vi "Vis-Prototype-ForceDirectedGraph-VIStaticLinkages.vi"() -> ()   [LabVIEW 2012]
uses:
  Dependencies/aws/AWS Shared/AWS-Shared-MetadataKeyValuePair.ctl
  Dependencies/aws/S3 API/AWS-S3-API.lvclass
panel:
  in  "Local Folder":path caption="(All output files will be copied to this location, old data may be overwritten!)"
  in  "Tab Control":T1(tab)=enum."HTML Page to Upload"
  in  "Local/Remote":string(combo)="Local"
  in  "S3 Bucket":string="visualize.wirebirdlabs.com" caption="(Default val provided merely as a convenience; feel free to output HTML/JSON to any local or remote server)"
  in  "Subfolder":string="gregSandbox" caption="(e.g., a subfolder \"mysandbox\" would upload to \"http://visualize.wirebirdlabs.com/mysandbox\")"
  in  "Access Key":string="AKIAJC4GLICEUISMCDHA"
  in  "Secret Key":string="WE0QzSnluCM5zp8GCpvH/PyVYhl7sW4CbsywKoKf"
  in  "Top-Level LabVIEW File (VI, LVClass, LVLib)":path caption="(e.g., drag the icon of this VI to this path control to scrape static linkages of itself)"
  in  "HTML Page":string="<!DOCTYPE HTML>\n<html dir=\"ltr\" lang=\"en-US\">\n\n<head>\n\n\t<!-- Title -->\n\t<title>VI Static Linkages as a Force-Directed Graph</title>\n\t\n\t<!-- SEO -->\n\t<meta name=\"robots\" content=\"noindex,noarchive,nosnippet\" />\n\n\t<!-- Stylesheets -->\n <link rel=\"stylesheet\" type=\"text/css\" media=\"all\" href=\"http://deploy.wirebirdlabs.com/Resources/Bootstrap/css/bootstrap.min.css\" />\n\t<link rel=\"stylesheet\" type=\"text/css\" media=\"all\" href=\"http://deploy.wirebirdlabs.com/Resources/FontAwesome/css/font-awesome.min.css\" />\n\t<link rel=\"stylesheet\" type=\"text/css\" media=\"all\" href=\"http://deploy.wirebirdlabs.com/Resources/Themes/Default/style.css\" />\n \n\t<!-- Scripts -->\n <script type='text/javascript' src='https://ajax.googleapis.com/ajax/libs/jquery/1.8.2/jquery.min.js'></script>\n\t<script type='text/javascript' src='http://deploy.wirebirdlabs.com/Resources/Bootstrap/js/bootstrap.min.js'></script>\n <script src=\"http://d3js.org/d3.v3.min.js\" charset=\"utf-8\"></script>\n\n\n <!-- Static Style Definitions -->\n <style>\n     .node {opacity: 0.5;}\n     .node:hover {opacity: 1;}\n     .node:not(:hover) text {display:none;}\n     .link {stroke: #999; stroke-opacity: 0.3;}\n</style>\n\n</head>\n\n<body class=\"container page-background\">\n\n\t<div class=\"container page-canvas\">\n\t\t<div class=\"page-header\">\n\t\t\t<h1 class=\"page-title page-title-title\">VI Static Linkages as a Force-Directed Graph</h1>\n\t\t</div>\n\n  <div class=\"page-body\">\n<div class=\"accordion\" id=\"legend\">\n  <div class=\"accordion-group template\">\n    <div class=\"accordion-heading\">\n        <a class=\"accordion-toggle\" data-toggle=\"collapse\" data-parent=\"#legend\" href=\"#collapseThree\">\n        </a>\n    </div>\n    <div id=\"collapseThree\" class=\"accordion-body collapse\">\n      <div class=\"accordion-inner\">\n      </div>\n    </div>\n  </div>\n</div>\n <!-- Begin code from http://bl.ocks.org/couchand/6420534 -->\n<div id=\"viz\"></div>\n <script>\n\nfunction name(d) { return d.name; }\nfunction group(d) { return d.group; }\n\nvar color = d3.scale.category10();\nfunction colorByGroup(d) { return color(group(d)); }\n\nvar width = <!-- Container-Width -->,\n    height = 960;\n\nvar svg = d3.select('#viz')\n    .append('svg')\n    .attr('width', width)\n    .attr('height', height);\n\nvar node, link;\n\nvar voronoi = d3.geom.voronoi()\n    .x(function(d) { return d.x; })\n    .y(function(d) { return d.y; })\n    .clipExtent([[-10, -10], [width+10, height+10]]);\n\nfunction recenterVoronoi(nodes) {\n    var shapes = [];\n    voronoi(nodes).forEach(function(d) {\n        if ( !d.length ) return;\n        var n = [];\n        d.forEach(function(c){\n            n.push([ c[0] - d.point.x, c[1] - d.point.y ]);\n        });\n        n.point = d.point;\n        shapes.push(n);\n    });\n    return shapes;\n}\n\nvar force = d3.layout.force()\n    .charge(-2000)\n    .friction(0.3)\n    .linkDistance(50)\n    .size([width, height]);\n\nforce.on('tick', function() {\n    node.attr('transform', function(d) { return 'translate('+d.x+','+d.y+')'; })\n        .attr('clip-path', function(d) { return 'url(#clip-'+d.index+')'; });\n\n    link.attr('x1', function(d) { return d.source.x; })\n        .attr('y1', function(d) { return d.source.y; })\n        .attr('x2', function(d) { return d.target.x; })\n        .attr('y2', function(d) { return d.target.y; });\n\n    var clip = svg.selectAll('.clip')\n        .data( recenterVoronoi(node.data()), function(d) { return d.point.index; } );\n\n    clip.enter().append('clipPath')\n        .attr('id', function(d) { return 'clip-'+d.point.index; })\n        .attr('class', 'clip');\n    clip.exit().remove()\n\n    clip.selectAll('path').remove();\n    clip.append('path')\n        .attr('d', function(d) { return 'M'+d.join(',')+'Z'; });\n});\n\nd3.json('root/static-linkages.json', function(err, data) {\n\n    data.nodes.forEach(function(d, i) {\n        d.id = i;\n    });\n\n    link = svg.selectAll('.link')\n        .data( data.links )\n      .enter().append('line')\n        .attr('class', 'link')\n        .style(\"stroke-width\", function(d) { return Math.sqrt(d.value); });\n\n    node = svg.selectAll('.node')\n        .data( data.nodes )\n      .enter().append('g')\n        .attr('title', name)\n        .attr('class', 'node')\n        .call( force.drag );\n\n    node.append('circle')\n        .attr('r', 30)\n        .attr('fill', colorByGroup)\n        .attr('fill-opacity', 0.5);\n\n    node.append('circle')\n        .attr('r', 4)\n        .attr('stroke', 'black');\n\n    node.append('text')\n        .text(function(d){return d.name;});\n\n    force\n        .nodes( data.nodes )\n        .links( data.links )\n        .start();\n\n\nvar $template = $(\".template\");\nvar names = new Array();\nnames = data.nodes;\nvar groupList = new Array();\n\n    function sortByKey(array, key) {\n    return array.sort(function(a, b) {\n        var x = a[key]; var y = b[key];\n        return ((x < y) ? -1 : ((x > y) ? 1 : 0));\n    });\n}\n\nsortByKey(names,'group');\n$.each(names, function(i,name) {\n    if (name.group != null && groupList.indexOf(name.group) < 0){\n    var $newPanel = $template.clone();\n    $newPanel.find(\".collapse\").removeClass(\"in\");\n    $newPanel.find(\".accordion-toggle\").attr(\"href\",  \"#\" + (name.group))\n             .text(\"Group #\" + name.group);\n    $newPanel.find(\".accordion-body\").attr(\"id\", name.group).addClass(\"collapse\").removeClass(\"in\");\n    $(\"#legend\").append($newPanel.fadeIn());\n    groupList.push(name.group);\n    }  \n$('#' + name.group).find('.accordion-inner').append(\"<p>\" + name.name + \"</p>\");\n});\n\nvar sortedLists;\n$.each(groupList,function(i,group){\n    var paragraphContent = $('#' + group).find('.accordion-inner p').get();\n    sortedLists = paragraphContent.sort(function(a, b){return ($(b).text().toUpperCase()) < ($(a).text().toUpperCase()) ? 1 : -1;})\n    $('#' + group).find('.accordion-inner').append(sortedLists);})\n\n});\n\n    </script>\n <!-- End code from http://bl.ocks.org/couchand/6420534 -->\n\n\t\t  <div class=\"page-footer row-fluid\">\n\t\t   \t<span class=\"span12\"></span>\n\t\t  </div>\n  </div>\n\t</div>\n\n\t<footer class=\"\">\n\t\t<p class=\"page-copyright\">Powered by: Friday nites and Halloween candy</p>\n\t\t<!-- Bootstrap Scripts -->\n\t\t<script type='text/javascript'>\n\t\t\tjQuery(document).ready( function(){\n\t\t\t\tjQuery('*[rel=popover]').popover();\n\t\t\t\tjQuery('*[rel=tooltip]').tooltip();} );\n\t\t</script>\n\t</footer>\n</body>\n</html>"
  in  "Default Data from http://bl.ocks.org/couchand/6420534":string="{\n  \"nodes\":[\n    {\"name\":\"Myriel\",\"group\":1},\n    {\"name\":\"Napoleon\",\"group\":1},\n    {\"name\":\"Mlle.Baptistine\",\"group\":1},\n    {\"name\":\"Mme.Magloire\",\"group\":1},\n    {\"name\":\"CountessdeLo\",\"group\":1},\n    {\"name\":\"Geborand\",\"group\":1},\n    {\"name\":\"Champtercier\",\"group\":1},\n    {\"name\":\"Cravatte\",\"group\":1},\n    {\"name\":\"Count\",\"group\":1},\n    {\"name\":\"OldMan\",\"group\":1},\n    {\"name\":\"Labarre\",\"group\":2},\n    {\"name\":\"Valjean\",\"group\":2},\n    {\"name\":\"Marguerite\",\"group\":3},\n    {\"name\":\"Mme.deR\",\"group\":2},\n    {\"name\":\"Isabeau\",\"group\":2},\n    {\"name\":\"Gervais\",\"group\":2},\n    {\"name\":\"Tholomyes\",\"group\":3},\n    {\"name\":\"Listolier\",\"group\":3},\n    {\"name\":\"Fameuil\",\"group\":3},\n    {\"name\":\"Blacheville\",\"group\":3},\n    {\"name\":\"Favourite\",\"group\":3},\n    {\"name\":\"Dahlia\",\"group\":3},\n    {\"name\":\"Zephine\",\"group\":3},\n    {\"name\":\"Fantine\",\"group\":3},\n    {\"name\":\"Mme.Thenardier\",\"group\":4},\n    {\"name\":\"Thenardier\",\"group\":4},\n    {\"name\":\"Cosette\",\"group\":5},\n    {\"name\":\"Javert\",\"group\":4},\n    {\"name\":\"Fauchelevent\",\"group\":0},\n    {\"name\":\"Bamatabois\",\"group\":2},\n    {\"name\":\"Perpetue\",\"group\":3},\n    {\"name\":\"Simplice\",\"group\":2},\n    {\"name\":\"Scaufflaire\",\"group\":2},\n    {\"name\":\"Woman1\",\"group\":2},\n    {\"name\":\"Judge\",\"group\":2},\n    {\"name\":\"Champmathieu\",\"group\":2},\n    {\"name\":\"Brevet\",\"group\":2},\n    {\"name\":\"Chenildieu\",\"group\":2},\n    {\"name\":\"Cochepaille\",\"group\":2},\n    {\"name\":\"Pontmercy\",\"group\":4},\n    {\"name\":\"Boulatruelle\",\"group\":6},\n    {\"name\":\"Eponine\",\"group\":4},\n    {\"name\":\"Anzelma\",\"group\":4},\n    {\"name\":\"Woman2\",\"group\":5},\n    {\"name\":\"MotherInnocent\",\"group\":0},\n    {\"name\":\"Gribier\",\"group\":0},\n    {\"name\":\"Jondrette\",\"group\":7},\n    {\"name\":\"Mme.Burgon\",\"group\":7},\n    {\"name\":\"Gavroche\",\"group\":8},\n    {\"name\":\"Gillenormand\",\"group\":5},\n    {\"name\":\"Magnon\",\"group\":5},\n    {\"name\":\"Mlle.Gillenormand\",\"group\":5},\n    {\"name\":\"Mme.Pontmercy\",\"group\":5},\n    {\"name\":\"Mlle.Vaubois\",\"group\":5},\n    {\"name\":\"Lt.Gillenormand\",\"group\":5},\n    {\"name\":\"Marius\",\"group\":8},\n    {\"name\":\"BaronessT\",\"group\":5},\n    {\"name\":\"Mabeuf\",\"group\":8},\n    {\"name\":\"Enjolras\",\"group\":8},\n    {\"name\":\"Combeferre\",\"group\":8},\n    {\"name\":\"Prouvaire\",\"group\":8},\n    {\"name\":\"Feuilly\",\"group\":8},\n    {\"name\":\"Courfeyrac\",\"group\":8},\n    {\"name\":\"Bahorel\",\"group\":8},\n    {\"name\":\"Bossuet\",\"group\":8},\n    {\"name\":\"Joly\",\"group\":8},\n    {\"name\":\"Grantaire\",\"group\":8},\n    {\"name\":\"MotherPlutarch\",\"group\":9},\n    {\"name\":\"Gueulemer\",\"group\":4},\n    {\"name\":\"Babet\",\"group\":4},\n    {\"name\":\"Claquesous\",\"group\":4},\n    {\"name\":\"Montparnasse\",\"group\":4},\n    {\"name\":\"Toussaint\",\"group\":5},\n    {\"name\":\"Child1\",\"group\":10},\n    {\"name\":\"Child2\",\"group\":10},\n    {\"name\":\"Brujon\",\"group\":4},\n    {\"name\":\"Mme.Hucheloup\",\"group\":8}\n  ],\n  \"links\":[\n    {\"source\":1,\"target\":0,\"value\":1},\n    {\"source\":2,\"target\":0,\"value\":8},\n    {\"source\":3,\"target\":0,\"value\":10},\n    {\"source\":3,\"target\":2,\"value\":6},\n    {\"source\":4,\"target\":0,\"value\":1},\n    {\"source\":5,\"target\":0,\"value\":1},\n    {\"source\":6,\"target\":0,\"value\":1},\n    {\"source\":7,\"target\":0,\"value\":1},\n    {\"source\":8,\"target\":0,\"value\":2},\n    {\"source\":9,\"target\":0,\"value\":1},\n    {\"source\":11,\"target\":10,\"value\":1},\n    {\"source\":11,\"target\":3,\"value\":3},\n    {\"source\":11,\"target\":2,\"value\":3},\n    {\"source\":11,\"target\":0,\"value\":5},\n    {\"source\":12,\"target\":11,\"value\":1},\n    {\"source\":13,\"target\":11,\"value\":1},\n    {\"source\":14,\"target\":11,\"value\":1},\n    {\"source\":15,\"target\":11,\"value\":1},\n    {\"source\":17,\"target\":16,\"value\":4},\n    {\"source\":18,\"target\":16,\"value\":4},\n    {\"source\":18,\"target\":17,\"value\":4},\n    {\"source\":19,\"target\":16,\"value\":4},\n    {\"source\":19,\"target\":17,\"value\":4},\n    {\"source\":19,\"target\":18,\"value\":4},\n    {\"source\":20,\"target\":16,\"value\":3},\n    {\"source\":20,\"target\":17,\"value\":3},\n    {\"source\":20,\"target\":18,\"value\":3},\n    {\"source\":20,\"target\":19,\"value\":4},\n    {\"source\":21,\"target\":16,\"value\":3},\n    {\"source\":21,\"target\":17,\"value\":3},\n    {\"source\":21,\"target\":18,\"value\":3},\n    {\"source\":21,\"target\":19,\"value\":3},\n    {\"source\":21,\"target\":20,\"value\":5},\n    {\"source\":22,\"target\":16,\"value\":3},\n    {\"source\":22,\"target\":17,\"value\":3},\n    {\"source\":22,\"target\":18,\"value\":3},\n    {\"source\":22,\"target\":19,\"value\":3},\n    {\"source\":22,\"target\":20,\"value\":4},\n    {\"source\":22,\"target\":21,\"value\":4},\n    {\"source\":23,\"target\":16,\"value\":3},\n    {\"source\":23,\"target\":17,\"value\":3},\n    {\"source\":23,\"target\":18,\"value\":3},\n    {\"source\":23,\"target\":19,\"value\":3},\n    {\"source\":23,\"target\":20,\"value\":4},\n    {\"source\":23,\"target\":21,\"value\":4},\n    {\"source\":23,\"target\":22,\"value\":4},\n    {\"source\":23,\"target\":12,\"value\":2},\n    {\"source\":23,\"target\":11,\"value\":9},\n    {\"source\":24,\"target\":23,\"value\":2},\n    {\"source\":24,\"target\":11,\"value\":7},\n    {\"source\":25,\"target\":24,\"value\":13},\n    {\"source\":25,\"target\":23,\"value\":1},\n    {\"source\":25,\"target\":11,\"value\":12},\n    {\"source\":26,\"target\":24,\"value\":4},\n    {\"source\":26,\"target\":11,\"value\":31},\n    {\"source\":26,\"target\":16,\"value\":1},\n    {\"source\":26,\"target\":25,\"value\":1},\n    {\"source\":27,\"target\":11,\"value\":17},\n    {\"source\":27,\"target\":23,\"value\":5},\n    {\"source\":27,\"target\":25,\"value\":5},\n    {\"source\":27,\"target\":24,\"value\":1},\n    {\"source\":27,\"target\":26,\"value\":1},\n    {\"source\":28,\"target\":11,\"value\":8},\n    {\"source\":28,\"target\":27,\"value\":1},\n    {\"source\":29,\"target\":23,\"value\":1},\n    {\"source\":29,\"target\":27,\"value\":1},\n    {\"source\":29,\"target\":11,\"value\":2},\n    {\"source\":30,\"target\":23,\"value\":1},\n    {\"source\":31,\"target\":30,\"value\":2},\n    {\"source\":31,\"target\":11,\"value\":3},\n    {\"source\":31,\"target\":23,\"value\":2},\n    {\"source\":31,\"target\":27,\"value\":1},\n    {\"source\":32,\"target\":11,\"value\":1},\n    {\"source\":33,\"target\":11,\"value\":2},\n    {\"source\":33,\"target\":27,\"value\":1},\n    {\"source\":34,\"target\":11,\"value\":3},\n    {\"source\":34,\"target\":29,\"value\":2},\n    {\"source\":35,\"target\":11,\"value\":3},\n    {\"source\":35,\"target\":34,\"value\":3},\n    {\"source\":35,\"target\":29,\"value\":2},\n    {\"source\":36,\"target\":34,\"value\":2},\n    {\"source\":36,\"target\":35,\"value\":2},\n    {\"source\":36,\"target\":11,\"value\":2},\n    {\"source\":36,\"target\":29,\"value\":1},\n    {\"source\":37,\"target\":34,\"value\":2},\n    {\"source\":37,\"target\":35,\"value\":2},\n    {\"source\":37,\"target\":36,\"value\":2},\n    {\"source\":37,\"target\":11,\"value\":2},\n    {\"source\":37,\"target\":29,\"value\":1},\n    {\"source\":38,\"target\":34,\"value\":2},\n    {\"source\":38,\"target\":35,\"value\":2},\n    {\"source\":38,\"target\":36,\"value\":2},\n    {\"source\":38,\"target\":37,\"value\":2},\n    {\"source\":38,\"target\":11,\"value\":2},\n    {\"source\":38,\"target\":29,\"value\":1},\n    {\"source\":39,\"target\":25,\"value\":1},\n    {\"source\":40,\"target\":25,\"value\":1},\n    {\"source\":41,\"target\":24,\"value\":2},\n    {\"source\":41,\"target\":25,\"value\":3},\n    {\"source\":42,\"target\":41,\"value\":2},\n    {\"source\":42,\"target\":25,\"value\":2},\n    {\"source\":42,\"target\":24,\"value\":1},\n    {\"source\":43,\"target\":11,\"value\":3},\n    {\"source\":43,\"target\":26,\"value\":1},\n    {\"source\":43,\"target\":27,\"value\":1},\n    {\"source\":44,\"target\":28,\"value\":3},\n    {\"source\":44,\"target\":11,\"value\":1},\n    {\"source\":45,\"target\":28,\"value\":2},\n    {\"source\":47,\"target\":46,\"value\":1},\n    {\"source\":48,\"target\":47,\"value\":2},\n    {\"source\":48,\"target\":25,\"value\":1},\n    {\"source\":48,\"target\":27,\"value\":1},\n    {\"source\":48,\"target\":11,\"value\":1},\n    {\"source\":49,\"target\":26,\"value\":3},\n    {\"source\":49,\"target\":11,\"value\":2},\n    {\"source\":50,\"target\":49,\"value\":1},\n    {\"source\":50,\"target\":24,\"value\":1},\n    {\"source\":51,\"target\":49,\"value\":9},\n    {\"source\":51,\"target\":26,\"value\":2},\n    {\"source\":51,\"target\":11,\"value\":2},\n    {\"source\":52,\"target\":51,\"value\":1},\n    {\"source\":52,\"target\":39,\"value\":1},\n    {\"source\":53,\"target\":51,\"value\":1},\n    {\"source\":54,\"target\":51,\"value\":2},\n    {\"source\":54,\"target\":49,\"value\":1},\n    {\"source\":54,\"target\":26,\"value\":1},\n    {\"source\":55,\"target\":51,\"value\":6},\n    {\"source\":55,\"target\":49,\"value\":12},\n    {\"source\":55,\"target\":39,\"value\":1},\n    {\"source\":55,\"target\":54,\"value\":1},\n    {\"source\":55,\"target\":26,\"value\":21},\n    {\"source\":55,\"target\":11,\"value\":19},\n    {\"source\":55,\"target\":16,\"value\":1},\n    {\"source\":55,\"target\":25,\"value\":2},\n    {\"source\":55,\"target\":41,\"value\":5},\n    {\"source\":55,\"target\":48,\"value\":4},\n    {\"source\":56,\"target\":49,\"value\":1},\n    {\"source\":56,\"target\":55,\"value\":1},\n    {\"source\":57,\"target\":55,\"value\":1},\n    {\"source\":57,\"target\":41,\"value\":1},\n    {\"source\":57,\"target\":48,\"value\":1},\n    {\"source\":58,\"target\":55,\"value\":7},\n    {\"source\":58,\"target\":48,\"value\":7},\n    {\"source\":58,\"target\":27,\"value\":6},\n    {\"source\":58,\"target\":57,\"value\":1},\n    {\"source\":58,\"target\":11,\"value\":4},\n    {\"source\":59,\"target\":58,\"value\":15},\n    {\"source\":59,\"target\":55,\"value\":5},\n    {\"source\":59,\"target\":48,\"value\":6},\n    {\"source\":59,\"target\":57,\"value\":2},\n    {\"source\":60,\"target\":48,\"value\":1},\n    {\"source\":60,\"target\":58,\"value\":4},\n    {\"source\":60,\"target\":59,\"value\":2},\n    {\"source\":61,\"target\":48,\"value\":2},\n    {\"source\":61,\"target\":58,\"value\":6},\n    {\"source\":61,\"target\":60,\"value\":2},\n    {\"source\":61,\"target\":59,\"value\":5},\n    {\"source\":61,\"target\":57,\"value\":1},\n    {\"source\":61,\"target\":55,\"value\":1},\n    {\"source\":62,\"target\":55,\"value\":9},\n    {\"source\":62,\"target\":58,\"value\":17},\n    {\"source\":62,\"target\":59,\"value\":13},\n    {\"source\":62,\"target\":48,\"value\":7},\n    {\"source\":62,\"target\":57,\"value\":2},\n    {\"source\":62,\"target\":41,\"value\":1},\n    {\"source\":62,\"target\":61,\"value\":6},\n    {\"source\":62,\"target\":60,\"value\":3},\n    {\"source\":63,\"target\":59,\"value\":5},\n    {\"source\":63,\"target\":48,\"value\":5},\n    {\"source\":63,\"target\":62,\"value\":6},\n    {\"source\":63,\"target\":57,\"value\":2},\n    {\"source\":63,\"target\":58,\"value\":4},\n    {\"source\":63,\"target\":61,\"value\":3},\n    {\"source\":63,\"target\":60,\"value\":2},\n    {\"source\":63,\"target\":55,\"value\":1},\n    {\"source\":64,\"target\":55,\"value\":5},\n    {\"source\":64,\"target\":62,\"value\":12},\n    {\"source\":64,\"target\":48,\"value\":5},\n    {\"source\":64,\"target\":63,\"value\":4},\n    {\"source\":64,\"target\":58,\"value\":10},\n    {\"source\":64,\"target\":61,\"value\":6},\n    {\"source\":64,\"target\":60,\"value\":2},\n    {\"source\":64,\"target\":59,\"value\":9},\n    {\"source\":64,\"target\":57,\"value\":1},\n    {\"source\":64,\"target\":11,\"value\":1},\n    {\"source\":65,\"target\":63,\"value\":5},\n    {\"source\":65,\"target\":64,\"value\":7},\n    {\"source\":65,\"target\":48,\"value\":3},\n    {\"source\":65,\"target\":62,\"value\":5},\n    {\"source\":65,\"target\":58,\"value\":5},\n    {\"source\":65,\"target\":61,\"value\":5},\n    {\"source\":65,\"target\":60,\"value\":2},\n    {\"source\":65,\"target\":59,\"value\":5},\n    {\"source\":65,\"target\":57,\"value\":1},\n    {\"source\":65,\"target\":55,\"value\":2},\n    {\"source\":66,\"target\":64,\"value\":3},\n    {\"source\":66,\"target\":58,\"value\":3},\n    {\"source\":66,\"target\":59,\"value\":1},\n    {\"source\":66,\"target\":62,\"value\":2},\n    {\"source\":66,\"target\":65,\"value\":2},\n    {\"source\":66,\"target\":48,\"value\":1},\n    {\"source\":66,\"target\":63,\"value\":1},\n    {\"source\":66,\"target\":61,\"value\":1},\n    {\"source\":66,\"target\":60,\"value\":1},\n    {\"source\":67,\"target\":57,\"value\":3},\n    {\"source\":68,\"target\":25,\"value\":5},\n    {\"source\":68,\"target\":11,\"value\":1},\n    {\"source\":68,\"target\":24,\"value\":1},\n    {\"source\":68,\"target\":27,\"value\":1},\n    {\"source\":68,\"target\":48,\"value\":1},\n    {\"source\":68,\"target\":41,\"value\":1},\n    {\"source\":69,\"target\":25,\"value\":6},\n    {\"source\":69,\"target\":68,\"value\":6},\n    {\"source\":69,\"target\":11,\"value\":1},\n    {\"source\":69,\"target\":24,\"value\":1},\n    {\"source\":69,\"target\":27,\"value\":2},\n    {\"source\":69,\"target\":48,\"value\":1},\n    {\"source\":69,\"target\":41,\"value\":1},\n    {\"source\":70,\"target\":25,\"value\":4},\n    {\"source\":70,\"target\":69,\"value\":4},\n    {\"source\":70,\"target\":68,\"value\":4},\n    {\"source\":70,\"target\":11,\"value\":1},\n    {\"source\":70,\"target\":24,\"value\":1},\n    {\"source\":70,\"target\":27,\"value\":1},\n    {\"source\":70,\"target\":41,\"value\":1},\n    {\"source\":70,\"target\":58,\"value\":1},\n    {\"source\":71,\"target\":27,\"value\":1},\n    {\"source\":71,\"target\":69,\"value\":2},\n    {\"source\":71,\"target\":68,\"value\":2},\n    {\"source\":71,\"target\":70,\"value\":2},\n    {\"source\":71,\"target\":11,\"value\":1},\n    {\"source\":71,\"target\":48,\"value\":1},\n    {\"source\":71,\"target\":41,\"value\":1},\n    {\"source\":71,\"target\":25,\"value\":1},\n    {\"source\":72,\"target\":26,\"value\":2},\n    {\"source\":72,\"target\":27,\"value\":1},\n    {\"source\":72,\"target\":11,\"value\":1},\n    {\"source\":73,\"target\":48,\"value\":2},\n    {\"source\":74,\"target\":48,\"value\":2},\n    {\"source\":74,\"target\":73,\"value\":3},\n    {\"source\":75,\"target\":69,\"value\":3},\n    {\"source\":75,\"target\":68,\"value\":3},\n    {\"source\":75,\"target\":25,\"value\":3},\n    {\"source\":75,\"target\":48,\"value\":1},\n    {\"source\":75,\"target\":41,\"value\":1},\n    {\"source\":75,\"target\":70,\"value\":1},\n    {\"source\":75,\"target\":71,\"value\":1},\n    {\"source\":76,\"target\":64,\"value\":1},\n    {\"source\":76,\"target\":65,\"value\":1},\n    {\"source\":76,\"target\":66,\"value\":1},\n    {\"source\":76,\"target\":63,\"value\":1},\n    {\"source\":76,\"target\":62,\"value\":1},\n    {\"source\":76,\"target\":48,\"value\":1},\n    {\"source\":76,\"target\":58,\"value\":1}\n  ]\n}"
  out "Status":string="Progress: 0049 of 0049"
  out "Nodes and Linkages":string="{\n\"nodes\":\n[    {\"name\":\"Vis-Prototype-ForceDirectedGraph-VIStaticLinkages.vi\",\"group\":2},\n     {\"name\":\"AWS-Shared-MetadataKeyValuePair.ctl\",\"group\":2},\n     {\"name\":\"WirebirdLabs-VIServer-LinkerInfo.vi\",\"group\":2},\n     {\"name\":\"WirebirdLabs-VIServer-LinkerInfoStructure.ctl\",\"group\":2},\n     {\"name\":\"FTW-JSON-Array-Serialize.vi\",\"group\":2},\n     {\"name\":\"WirebirdLabs-STR-DelimitStringArray.vi\",\"group\":2},\n     {\"name\":\"AWS-S3-API.lvclass:AWS-S3-ConstructClient.vi\",\"group\":1},\n     {\"name\":\"AWS-S3-API.lvclass\",\"group\":0},\n     {\"name\":\"AWS-S3-API.lvclass:AWS-S3-API.ctl\",\"group\":1},\n     {\"name\":\"mscorlib\",\"group\":4},\n     {\"name\":\"AWS-S3-API.lvclass:AWS-S3-Transfer-Progress.ctl\",\"group\":1},\n     {\"name\":\"AWS-S3-API.lvclass:AWS-S3-Transfer-Header.ctl\",\"group\":1},\n     {\"name\":\"AWS-S3-API.lvclass:AWS-S3-Transfer-Completed.ctl\",\"group\":1},\n     {\"name\":\"AWS-S3-API.lvclass:AWS-S3-ClientRef-Get.vi\",\"group\":1},\n     {\"name\":\"E:\\u005CWirebirdLabs\\u005CVisualize\\u005CDependencies\\u005Caws\\u005CAWS-SDK\\u005CAWSSDK.dll\",\"group\":4},\n     {\"name\":\"AWS-S3-API.lvclass:AWS-S3-ClientRef-Set.vi\",\"group\":1},\n     {\"name\":\"AWS-S3-API.lvclass:AWS-S3-ObjectURL.vi\",\"group\":1},\n     {\"name\":\"WirebirdLabs-ERR-Clear.vi\",\"group\":2},\n     {\"name\":\"AWS-S3-API.lvclass:AWS-S3-ProcessDownload.vi\",\"group\":1},\n     {\"name\":\"AWS-S3-API.lvclass:AWS-S3-ProcessUpload.vi\",\"group\":1},\n     {\"name\":\"AWS-S3-API.lvclass:AWS-S3-ProgressCallbackDownload.vi\",\"group\":1},\n     {\"name\":\"AWS-S3-API.lvclass:AWS-S3-SendProgressUpdate.vi\",\"group\":1},\n     {\"name\":\"AWS-S3-API.lvclass:AWS-S3-ProgressCallbackUpload.vi\",\"group\":1},\n     {\"name\":\"AWS-S3-API.lvclass:AWS-S3-BeginDownload.vi\",\"group\":1},\n     {\"name\":\"WirebirdLabs-Time-Timer.vi\",\"group\":2},\n     {\"name\":\"WirebirdLabs-VIServer-AsyncCallOptions.vi\",\"group\":2},\n     {\"name\":\"AWS-S3-API.lvclass:AWS-S3-BeginUpload.vi\",\"group\":1},\n     {\"name\":\"WirebirdLabs-File-FileInfo.vi\",\"group\":2},\n     {\"name\":\"FTW-STR-Display-Bytes.vi\",\"group\":2},\n     {\"name\":\"AWS-Shared-MD5ofFile.vi\",\"group\":2},\n     {\"name\":\"AWS-S3-API.lvclass:AWS-S3-BucketCreate.vi\",\"group\":1},\n     {\"name\":\"AWS-S3-API.lvclass:AWS-S3-BucketSetPolicy.vi\",\"group\":1},\n     {\"name\":\"AWS-S3-API.lvclass:AWS-S3-BucketSettings.vi\",\"group\":1},\n     {\"name\":\"AWS-S3-API.lvclass:AWS-S3-DestroyClient.vi\",\"group\":1},\n     {\"name\":\"AWS-S3-API.lvclass:AWS-S3-GenerateExpiringLink.vi\",\"group\":1},\n     {\"name\":\"AWS-S3-API.lvclass:AWS-S3-GetObjectData.vi\",\"group\":1},\n     {\"name\":\"AWS-S3-API.lvclass:AWS-S3-GetProgressEvent.vi\",\"group\":1},\n     {\"name\":\"AWS-S3-API.lvclass:AWS-S3-ListBuckets.vi\",\"group\":1},\n     {\"name\":\"AWS-S3-API.lvclass:AWS-S3-ListObjectsInBucket.vi\",\"group\":1},\n     {\"name\":\"System\",\"group\":4},\n     {\"name\":\"AWS-S3-API.lvclass:AWS-S3-PutObjectData.vi\",\"group\":1},\n     {\"name\":\"AWS-Shared-MD5ofContent.vi\",\"group\":2},\n     {\"name\":\"AWS-S3-API.lvclass:AWS-S3-SynchronousUpload.vi\",\"group\":1},\n     {\"name\":\"AWS-S3-API.lvclass:AWS-S3-Transfer-Abort.vi\",\"group\":1},\n     {\"name\":\"Get File Extension.vi\",\"group\":2},\n     {\"name\":\"C:\\u005CProgram Files (x86)\\u005CNational Instruments\\u005CLabVIEW 2012\\u005Chelp\\u005Cglang.chm\",\"group\":4},\n     {\"name\":\"FTW-JSON-Format-String.vi\",\"group\":2},\n     {\"name\":\"WirebirdLabs-JSON-Escape.vi\",\"group\":2},\n     {\"name\":\"Error Cluster From Error Code.vi\",\"group\":2}],\n\"links\":\n[    {\"source\":0,\"target\":1,\"value\":9},\n     {\"source\":0,\"target\":2,\"value\":9},\n     {\"source\":0,\"target\":4,\"value\":9},\n     {\"source\":0,\"target\":6,\"value\":9},\n     {\"source\":0,\"target\":40,\"value\":9},\n     {\"source\":0,\"target\":33,\"value\":9},\n     {\"source\":0,\"target\":44,\"value\":9},\n     {\"source\":0,\"target\":46,\"value\":9},\n     {\"source\":0,\"target\":48,\"value\":9},\n     {\"source\":2,\"target\":3,\"value\":1},\n     {\"source\":4,\"target\":5,\"value\":1},\n     {\"source\":6,\"target\":7,\"value\":7},\n     {\"source\":6,\"target\":10,\"value\":7},\n     {\"source\":6,\"target\":11,\"value\":7},\n     {\"source\":6,\"target\":12,\"value\":7},\n     {\"source\":6,\"target\":14,\"value\":7},\n     {\"source\":6,\"target\":8,\"value\":7},\n     {\"source\":6,\"target\":15,\"value\":7},\n     {\"source\":7,\"target\":8,\"value\":27},\n     {\"source\":7,\"target\":13,\"value\":27},\n     {\"source\":7,\"target\":15,\"value\":27},\n     {\"source\":7,\"target\":16,\"value\":27},\n     {\"source\":7,\"target\":18,\"value\":27},\n     {\"source\":7,\"target\":19,\"value\":27},\n     {\"source\":7,\"target\":20,\"value\":27},\n     {\"source\":7,\"target\":22,\"value\":27},\n     {\"source\":7,\"target\":21,\"value\":27},\n     {\"source\":7,\"target\":23,\"value\":27},\n     {\"source\":7,\"target\":26,\"value\":27},\n     {\"source\":7,\"target\":30,\"value\":27},\n     {\"source\":7,\"target\":31,\"value\":27},\n     {\"source\":7,\"target\":32,\"value\":27},\n     {\"source\":7,\"target\":6,\"value\":27},\n     {\"source\":7,\"target\":33,\"value\":27},\n     {\"source\":7,\"target\":34,\"value\":27},\n     {\"source\":7,\"target\":35,\"value\":27},\n     {\"source\":7,\"target\":36,\"value\":27},\n     {\"source\":7,\"target\":37,\"value\":27},\n     {\"source\":7,\"target\":38,\"value\":27},\n     {\"source\":7,\"target\":40,\"value\":27},\n     {\"source\":7,\"target\":42,\"value\":27},\n     {\"source\":7,\"target\":43,\"value\":27},\n     {\"source\":7,\"target\":12,\"value\":27},\n     {\"source\":7,\"target\":11,\"value\":27},\n     {\"source\":7,\"target\":10,\"value\":27},\n     {\"source\":8,\"target\":7,\"value\":5},\n     {\"source\":8,\"target\":9,\"value\":5},\n     {\"source\":8,\"target\":10,\"value\":5},\n     {\"source\":8,\"target\":11,\"value\":5},\n     {\"source\":8,\"target\":12,\"value\":5},\n     {\"source\":10,\"target\":7,\"value\":2},\n     {\"source\":10,\"target\":11,\"value\":2},\n     {\"source\":11,\"target\":7,\"value\":1},\n     {\"source\":12,\"target\":7,\"value\":2},\n     {\"source\":12,\"target\":11,\"value\":2},\n     {\"source\":13,\"target\":7,\"value\":3},\n     {\"source\":13,\"target\":14,\"value\":3},\n     {\"source\":13,\"target\":8,\"value\":3},\n     {\"source\":15,\"target\":7,\"value\":3},\n     {\"source\":15,\"target\":14,\"value\":3},\n     {\"source\":15,\"target\":8,\"value\":3},\n     {\"source\":16,\"target\":7,\"value\":2},\n     {\"source\":16,\"target\":17,\"value\":2},\n     {\"source\":18,\"target\":7,\"value\":5},\n     {\"source\":18,\"target\":12,\"value\":5},\n     {\"source\":18,\"target\":11,\"value\":5},\n     {\"source\":18,\"target\":14,\"value\":5},\n     {\"source\":18,\"target\":17,\"value\":5},\n     {\"source\":19,\"target\":7,\"value\":5},\n     {\"source\":19,\"target\":14,\"value\":5},\n     {\"source\":19,\"target\":12,\"value\":5},\n     {\"source\":19,\"target\":11,\"value\":5},\n     {\"source\":19,\"target\":17,\"value\":5},\n     {\"source\":20,\"target\":7,\"value\":6},\n     {\"source\":20,\"target\":14,\"value\":6},\n     {\"source\":20,\"target\":9,\"value\":6},\n     {\"source\":20,\"target\":10,\"value\":6},\n     {\"source\":20,\"target\":11,\"value\":6},\n     {\"source\":20,\"target\":21,\"value\":6},\n     {\"source\":21,\"target\":7,\"value\":3},\n     {\"source\":21,\"target\":10,\"value\":3},\n     {\"source\":21,\"target\":11,\"value\":3},\n     {\"source\":22,\"target\":7,\"value\":6},\n     {\"source\":22,\"target\":14,\"value\":6},\n     {\"source\":22,\"target\":9,\"value\":6},\n     {\"source\":22,\"target\":10,\"value\":6},\n     {\"source\":22,\"target\":11,\"value\":6},\n     {\"source\":22,\"target\":21,\"value\":6},\n     {\"source\":23,\"target\":7,\"value\":10},\n     {\"source\":23,\"target\":10,\"value\":10},\n     {\"source\":23,\"target\":11,\"value\":10},\n     {\"source\":23,\"target\":8,\"value\":10},\n     {\"source\":23,\"target\":14,\"value\":10},\n     {\"source\":23,\"target\":24,\"value\":10},\n     {\"source\":23,\"target\":25,\"value\":10},\n     {\"source\":23,\"target\":18,\"value\":10},\n     {\"source\":23,\"target\":20,\"value\":10},\n     {\"source\":23,\"target\":13,\"value\":10},\n     {\"source\":26,\"target\":7,\"value\":15},\n     {\"source\":26,\"target\":1,\"value\":15},\n     {\"source\":26,\"target\":10,\"value\":15},\n     {\"source\":26,\"target\":11,\"value\":15},\n     {\"source\":26,\"target\":8,\"value\":15},\n     {\"source\":26,\"target\":9,\"value\":15},\n     {\"source\":26,\"target\":14,\"value\":15},\n     {\"source\":26,\"target\":25,\"value\":15},\n     {\"source\":26,\"target\":19,\"value\":15},\n     {\"source\":26,\"target\":22,\"value\":15},\n     {\"source\":26,\"target\":16,\"value\":15},\n     {\"source\":26,\"target\":24,\"value\":15},\n     {\"source\":26,\"target\":27,\"value\":15},\n     {\"source\":26,\"target\":29,\"value\":15},\n     {\"source\":26,\"target\":13,\"value\":15},\n     {\"source\":27,\"target\":28,\"value\":1},\n     {\"source\":28,\"target\":17,\"value\":1},\n     {\"source\":29,\"target\":9,\"value\":2},\n     {\"source\":29,\"target\":14,\"value\":2},\n     {\"source\":30,\"target\":7,\"value\":3},\n     {\"source\":30,\"target\":14,\"value\":3},\n     {\"source\":30,\"target\":13,\"value\":3},\n     {\"source\":31,\"target\":7,\"value\":3},\n     {\"source\":31,\"target\":14,\"value\":3},\n     {\"source\":31,\"target\":13,\"value\":3},\n     {\"source\":32,\"target\":7,\"value\":3},\n     {\"source\":32,\"target\":14,\"value\":3},\n     {\"source\":32,\"target\":13,\"value\":3},\n     {\"source\":33,\"target\":7,\"value\":5},\n     {\"source\":33,\"target\":14,\"value\":5},\n     {\"source\":33,\"target\":8,\"value\":5},\n     {\"source\":33,\"target\":13,\"value\":5},\n     {\"source\":33,\"target\":17,\"value\":5},\n     {\"source\":34,\"target\":7,\"value\":3},\n     {\"source\":34,\"target\":14,\"value\":3},\n     {\"source\":34,\"target\":13,\"value\":3},\n     {\"source\":35,\"target\":7,\"value\":4},\n     {\"source\":35,\"target\":14,\"value\":4},\n     {\"source\":35,\"target\":9,\"value\":4},\n     {\"source\":35,\"target\":13,\"value\":4},\n     {\"source\":36,\"target\":7,\"value\":5},\n     {\"source\":36,\"target\":10,\"value\":5},\n     {\"source\":36,\"target\":11,\"value\":5},\n     {\"source\":36,\"target\":12,\"value\":5},\n     {\"source\":36,\"target\":8,\"value\":5},\n     {\"source\":37,\"target\":7,\"value\":4},\n     {\"source\":37,\"target\":14,\"value\":4},\n     {\"source\":37,\"target\":9,\"value\":4},\n     {\"source\":37,\"target\":13,\"value\":4},\n     {\"source\":38,\"target\":7,\"value\":5},\n     {\"source\":38,\"target\":14,\"value\":5},\n     {\"source\":38,\"target\":39,\"value\":5},\n     {\"source\":38,\"target\":9,\"value\":5},\n     {\"source\":38,\"target\":13,\"value\":5},\n     {\"source\":40,\"target\":7,\"value\":6},\n     {\"source\":40,\"target\":1,\"value\":6},\n     {\"source\":40,\"target\":14,\"value\":6},\n     {\"source\":40,\"target\":16,\"value\":6},\n     {\"source\":40,\"target\":13,\"value\":6},\n     {\"source\":40,\"target\":41,\"value\":6},\n     {\"source\":41,\"target\":14,\"value\":1},\n     {\"source\":42,\"target\":7,\"value\":4},\n     {\"source\":42,\"target\":1,\"value\":4},\n     {\"source\":42,\"target\":14,\"value\":4},\n     {\"source\":42,\"target\":13,\"value\":4},\n     {\"source\":43,\"target\":7,\"value\":5},\n     {\"source\":43,\"target\":8,\"value\":5},\n     {\"source\":43,\"target\":9,\"value\":5},\n     {\"source\":43,\"target\":14,\"value\":5},\n     {\"source\":43,\"target\":17,\"value\":5},\n     {\"source\":44,\"target\":45,\"value\":1},\n     {\"source\":46,\"target\":47,\"value\":1},\n     {\"source\":48,\"target\":45,\"value\":1}]\n}"
  out "error out":errorcluster
  # "var $template = $(\".template\");\nvar hash = 2;\nvar names = new Array();\nnames = data.nodes;\nvar groupList = new Array();\n\n    function sortByKey(array, key) {\n    return array.sort(function(a, b) {\n        var x = a[key]; var y = b[key];\n        return ((x < y) ? -1 : ((x > y) ? 1 : 0));\n    });\n}\nsortByKey(names,'group');\n$.each(names, function(i,name) {\n    if (name.group != null && groupList.indexOf(name.group) < 0){\n    var $newPanel = $template.clone();\n    $newPanel.find(\".collapse\").removeClass(\"in\");\n    $newPanel.find(\".accordion-toggle\").attr(\"href\",  \"#\" + (name.group))\n             .text(\"Group #\" + name.group);\n    $newPanel.find(\".panel-collapse\").attr(\"id\", name.group).addClass(\"collapse\").removeClass(\"in\");\n    $(\"#accordion\").append($newPanel.fadeIn());\n    groupList.push(name.group);\n    }  \n$('#' + name.group).find('.panel-body').append(\"<p>\" + name.name + \"</p>\");\n});\n\nvar sortedLists;\n$.each(groupList,function(i,group){\n    var paragraphContent = $('#' + group).find('.panel-body p').get();\n    sortedLists = paragraphContent.sort(function(a, b){return ($(b).text()) < ($(a).text()) ? 1 : -1;})\n    $('#' + group).find('.panel-body').append(sortedLists);})"
  # "<div class=\"panel-group\" id=\"accordion\">\n  <div class=\"panel panel-default template\">\n    <div class=\"panel-heading\">\n      <h4 class=\"panel-title\">\n        <a class=\"accordion-toggle\" data-toggle=\"collapse\" data-parent=\"#accordion\" href=\"#collapseThree\">\n        </a>\n      </h4>\n    </div>\n    <div id=\"collapseThree\" class=\"panel-collapse collapse\">\n      <div class=\"panel-body\">\n      </div>\n    </div>\n  </div>\n</div>"
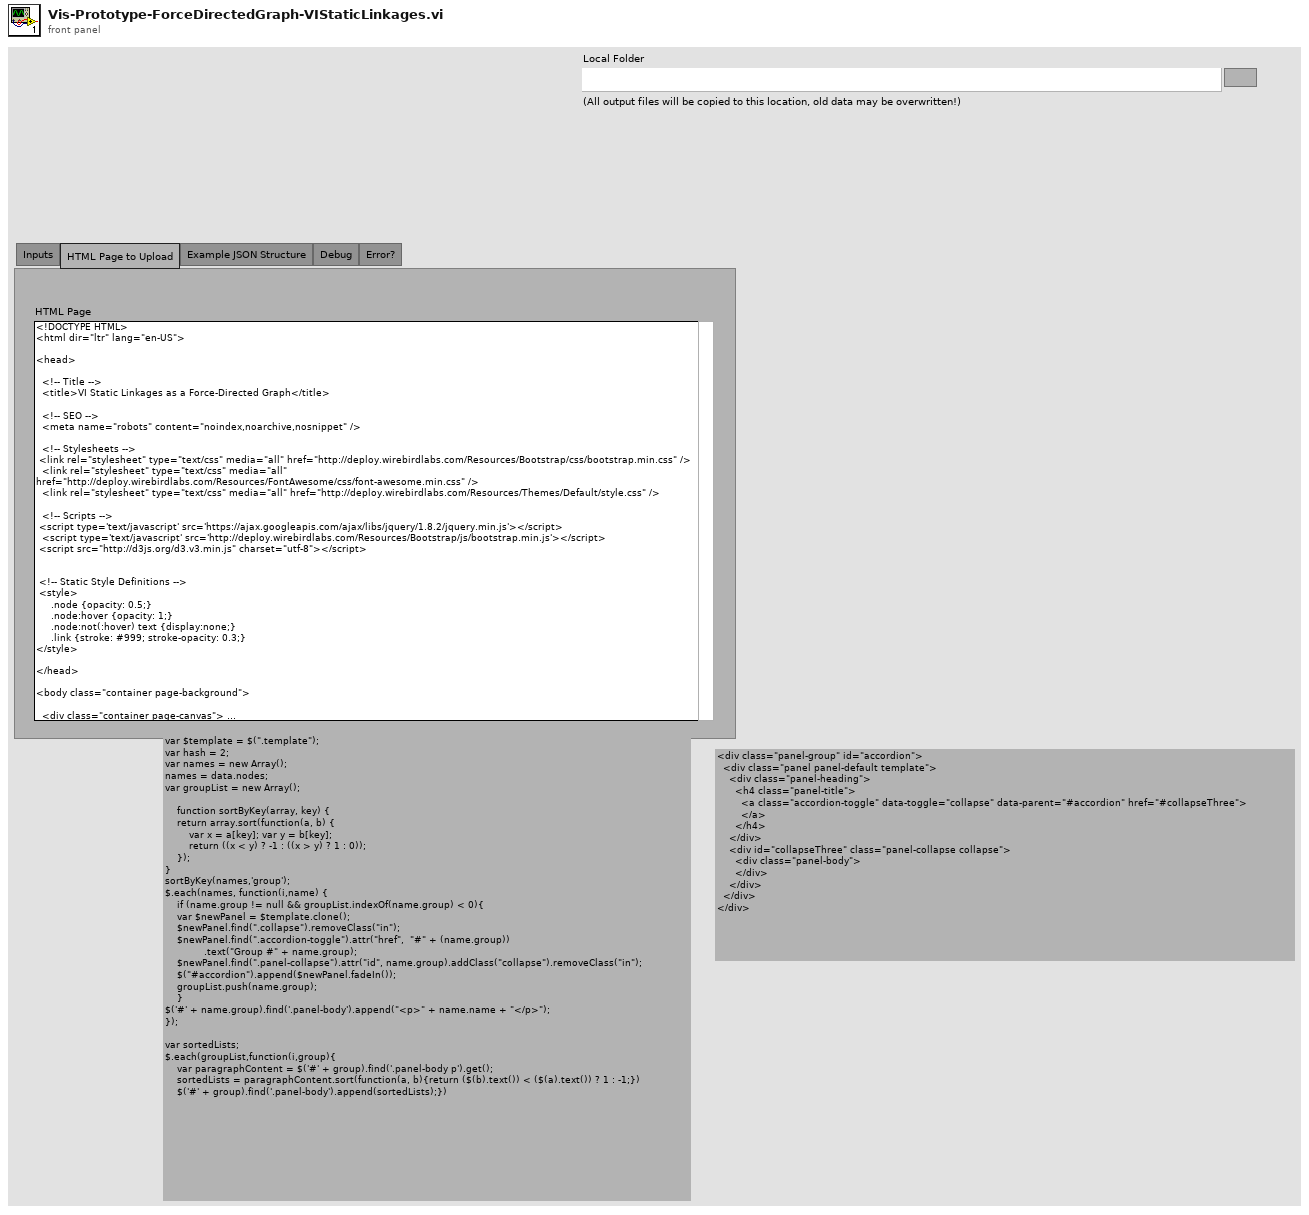
[diagram p1: front panel]
types:
  T1 = enum32{"Inputs", "HTML Page to Upload", "Example JSON Structure", "Debug", "Error?"}
  T2 = typedef "WirebirdLabs-VIServer-LinkerInfoStructure.ctl" = cluster{"path":path, "delimited name":string, "Filetype":string, "iState":u32, "iStyle":u16, "wStyle":u16, "buttons":u16, "viflags":u32, "viflags2":u32, "links":u32[]}
  T3 = typedef "AWS-Shared-MetadataKeyValuePair.ctl" = cluster{"Key":string, "Value":string}
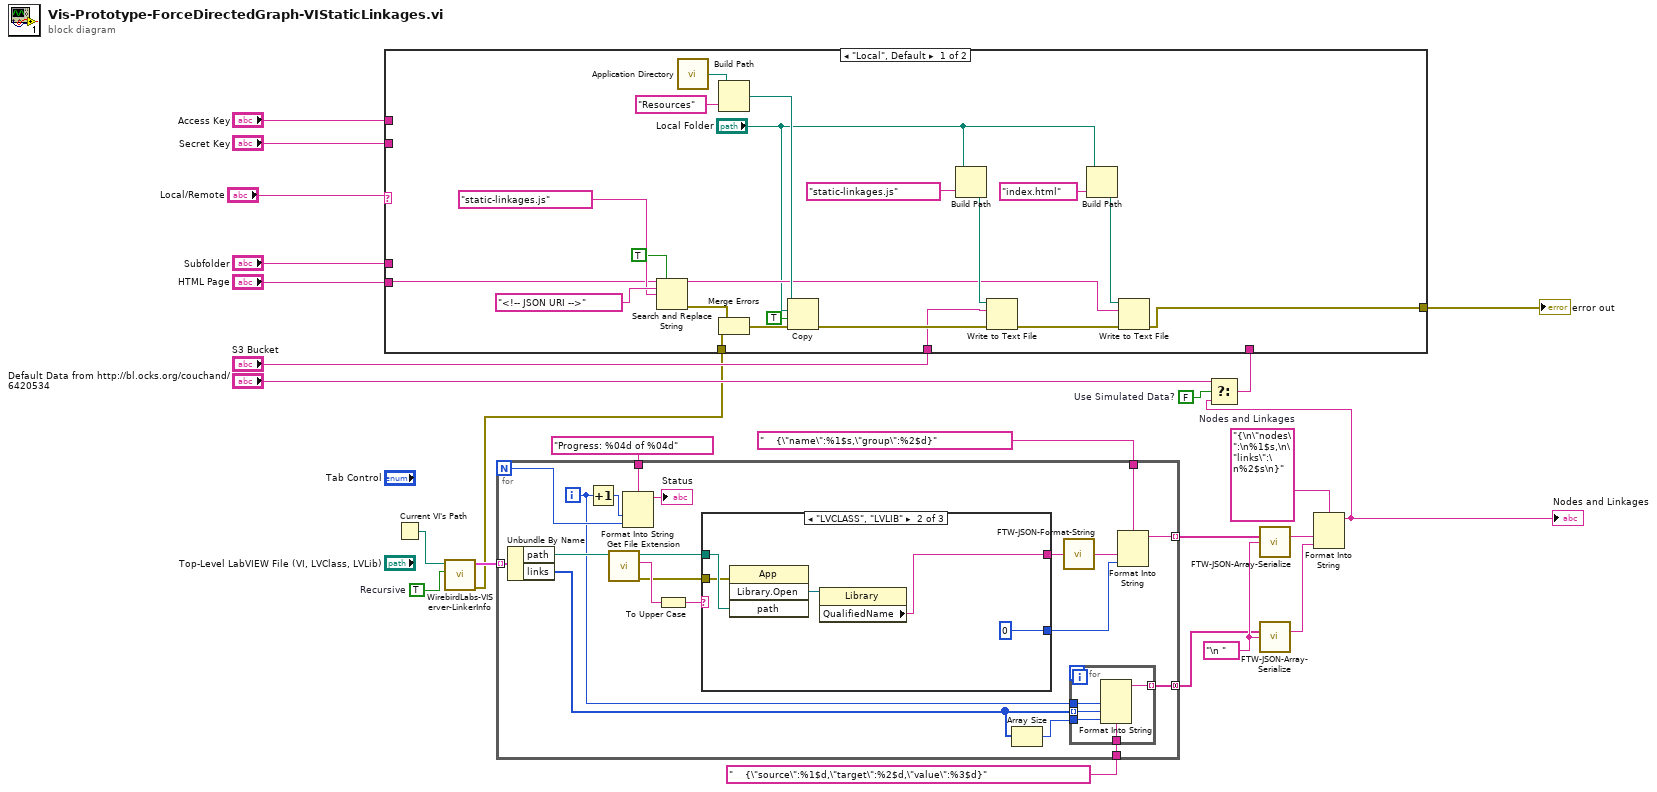
[diagram p0: block diagram]
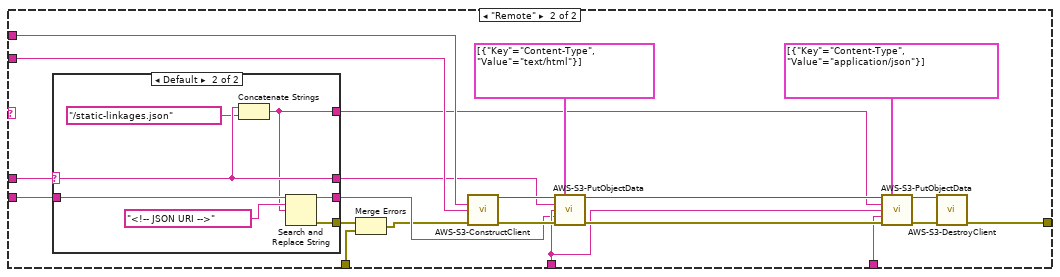
[diagram p2: hidden frame]
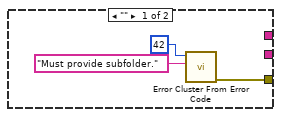
[diagram p3: hidden frame]
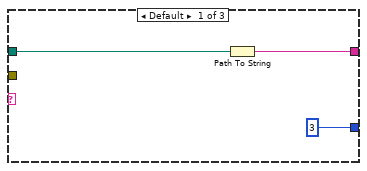
[diagram p4: hidden frame]
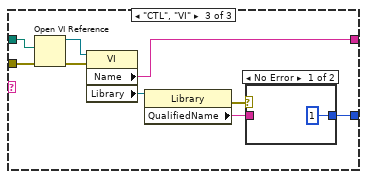
[diagram p5: hidden frame]
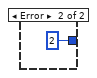
[diagram p6: hidden frame]
diagram:
  w11 = FALSE  # Use Simulated Data?
  w16 = "\n " ("Whitespace Delimiter (after commas)")
  w20 = "{\n\"nodes\":\n%1$s,\n\"links\":\n%2$s\n}"  # Nodes and Linkages
  w21 = TRUE  # Recursive
  n1 = Current VI's Path() -> (path=w2:path)
  n2 = call "WirebirdLabs-VIServer-LinkerInfo.vi"("Recursive"=w21, "LabVIEW Filetype"=w2) -> ("error out"=w3:errorcluster, "LinkerInfo"=w14:T2[])  [unwired: 8 in]
  n3 = for {
    N -> [w37]
    tunnel: w14 -> [w39] mode=indexing
    tunnel: [w27] -> w18 mode=indexing
    tunnel: "Progress: %04d of %04d" -> [w38]
    tunnel: [w34] -> w13 mode=concatenating
    tunnel: "    {\"name\":%1$s,\"group\":%2$d}" -> [w30]
    tunnel: "    {\"source\":%1$d,\"target\":%2$d,\"value\":%3$d}" -> [w25]
    i -> [w31]
    n4 = Unbundle By Name(w39) -> ("path"=w43:path, "links"=w33:u32[])
    n5 = Increment(x=w31) -> (x+1=w35:i32)
    n6 = call <vilib>:"Get File Extension.vi"("file"=w43) -> ("error out"=w40:errorcluster, "lowercase file extension"=w44:string, "dup file"=w42:path)  [unwired: 7 in, 1 out]
    n7 = Format Into String(format string=w38, w35, w37) -> (resulting string=→"Status":string)  [unwired: 2 in, 1 out]
    n8 = To Upper Case(1:w44) -> (0:w41:string)
    n9 = case shown="\"LVCLASS\", \"LVLIB\"" w41 {
      tunnel: w42 -> [w52 w57 w66]
      tunnel: w40 -> [_ w56 w62]
      tunnel: [w51 w54 w59] -> w28
      tunnel: [3 ("input 2") 0 ("input 2") w58] -> w26
      frame Default {
        n10 = Path To String(path=w52) -> (string=w51:string)
      }
      frame "LVCLASS", "LVLIB" {
        n11 = invoke class="App" method="Library.Open"(error in=w56, "path"=w57) -> ("Open Library"=w55:refnum<vi>)  [unwired: 2 in, 3 out]
        n12 = property class="Library"(reference=w55) -> ("QualifiedName"=w54:string)  [unwired: 1 in, 2 out]
      }
      frame "CTL", "VI" {
        n13 = Open VI Reference(vi path=w66, error in (no error)=w62) -> (vi reference=w65:refnum<vi>, error out=w64:errorcluster)  [unwired: 4 in]
        n14 = property class="VI"(reference=w65, error in=w64) -> ("Name"=w59:string, "Library"=w63:refnum<vi>)  [unwired: 2 out]
        n15 = property class="Library"(reference=w63) -> (error out=w61:errorcluster, "QualifiedName"=w60:string)  [unwired: 1 in, 1 out]
        n16 = case shown="No Error" w61 {
          tunnel: w60 -> [_ _]
          tunnel: [1 2] -> w58
          frame No Error {
          }
          frame Error {
          }
        }
      }
    }
    n17 = Array Size(array=w33) -> (size(s)=w32:i32)
    n18 = call "FTW-JSON-Format-String.vi"("LabVIEW String"=w28) -> ("JSON String"=w29:string)
    n19 = for {
      tunnel: w33 -> [w48] mode=indexing
      tunnel: w31 -> [w49]
      tunnel: [w47] -> w34 mode=indexing
      tunnel: w32 -> [w46]
      tunnel: w25 -> [w45]
      n20 = Format Into String(format string=w45, w49, w48, w46) -> (resulting string=w47:string)  [unwired: 2 in, 1 out]
    }
    n21 = Format Into String(format string=w30, w29, w26) -> (resulting string=w27:string)  [unwired: 2 in, 1 out]
  }
  n22 = call "FTW-JSON-Array-Serialize.vi"("Array of JSON Elements"=w18, "Whitespace Delimiter (after commas)"=w16) -> ("JSON Array"=w19:string)  [unwired: 13 in]
  n23 = call "FTW-JSON-Array-Serialize.vi"("Array of JSON Elements"=w13, "Whitespace Delimiter (after commas)"=w16) -> ("JSON Array"=w17:string)  [unwired: 13 in]
  n24 = Format Into String(format string=w20, w19, w17) -> (resulting string=w10:string)  [unwired: 2 in, 1 out]
  "Nodes and Linkages" <- w10
  n25 = Select(t="Default Data from http://bl.ocks.org/couchand/6420534", s=w11, f=w10) -> (s? t:f=w12:string)
  n26 = case shown="\"Local\", Default" "Local/Remote" {
    tunnel: [w69 w102] -> w24
    tunnel: "Access Key" -> [_ w101]
    tunnel: "Secret Key" -> [_ w100]
    tunnel: w12 -> [_ w99]
    tunnel: "Subfolder" -> [_ w98]
    tunnel: "S3 Bucket" -> [w70 w97]
    tunnel: "HTML Page" -> [w72 w94]
    tunnel: w3 -> [w71 w90]
    frame "Local", Default {
      n27 = Search and Replace String(replace all?=TRUE ("replace all? (F)"), input string=w72, search string="<!-- JSON URI -->", replace string="static-linkages.js" ("Object Key")) -> (result string=w79:string, error out=w80:errorcluster)  [unwired: 4 in, 2 out]
      n28 = call <vilib>:"Application Directory.vi"() -> ("Application Directory"=w89:path)
      n29 = Build Path(base path=w89, name or relative path="Resources" ("Object Key")) -> (appended path=w82:path)
      n30 = Merge Errors(w80, w71) -> (w88:errorcluster)
      n31 = Copy(8:w88, 9:TRUE ("overwrite (F)"), 10:"Local Folder", 11:w82) -> (0:w86:errorcluster)  [unwired: 1 in, 2 out]
      n32 = Build Path(base path="Local Folder", name or relative path="static-linkages.js" ("Object Key")) -> (appended path=w84:path)
      n33 = Write to Text File(file (use dialog)=w84, text=w70, error in=w86) -> (error out=w83:errorcluster)  [unwired: 1 in, 2 out]
      n34 = Build Path(base path="Local Folder", name or relative path="index.html" ("Object Key")) -> (appended path=w81:path)
      n35 = Write to Text File(file (use dialog)=w81, text=w79, error in=w83) -> (error out=w69:errorcluster)  [unwired: 1 in, 2 out]
    }
    frame "Remote" {
      n36 = case shown="Default" w98 {
        selector: w98 -> [_ w120]
        tunnel: [w113 w117] -> w92
        tunnel: [_ w120] -> w96
        tunnel: [_ w114] -> w95
        tunnel: w94 -> [_ w118]
        tunnel: [_ w116] -> w93
        frame "" {
          n37 = call <vilib>:"Error Cluster From Error Code.vi"("error message (\"\")"="Must provide subfolder." ("error message (\"\")"), "error code (0)"=42) -> ("error out"=w113:errorcluster)  [unwired: 7 in]
        }
        frame Default {
          n38 = Concatenate Strings(w120, "/static-linkages.json" ("Object Key")) -> (w114:string)
          n39 = Search and Replace String(input string=w118, search string="<!-- JSON URI -->", replace string=w114) -> (result string=w116:string, error out=w117:errorcluster)  [unwired: 5 in, 2 out]
        }
      }
      n40 = Merge Errors(w92, w90) -> (w91:errorcluster)
      n41 = call "AWS-S3-ConstructClient.vi"("Access Key"=w101, "Secret Key"=w100, "error in"=w91) -> ("AWS-S3-API"=w110:refnum<class "AWS-S3-API.lvclass">, "error out"=w109:errorcluster)  [unwired: 11 in]
      n42 = call "AWS-S3-PutObjectData.vi"("AWS-S3-API"=w110, "Headers"=T3[] [{"Key"="Content-Type", "Value"="text/html"}], "Object Key"=w96, "Object Bucket"=w97, "Object Data"=w93, "error in"=w109) -> ("AWS-S3-API out"=w108:refnum<class "AWS-S3-API.lvclass">, "error out"=w107:errorcluster)  [unwired: 6 in, 2 out]
      n43 = call "AWS-S3-PutObjectData.vi"("AWS-S3-API"=w108, "Headers"=T3[] [{"Key"="Content-Type", "Value"="application/json"}], "Object Key"=w95, "Object Bucket"=w97, "Object Data"=w99, "error in"=w107) -> ("AWS-S3-API out"=w106:refnum<class "AWS-S3-API.lvclass">, "error out"=w105:errorcluster)  [unwired: 6 in, 2 out]
      n44 = call "AWS-S3-DestroyClient.vi"("AWS-S3-API"=w106, "error in"=w105) -> ("error out"=w102:errorcluster)  [unwired: 13 in]
    }
  }
  "error out" <- w24
